vi "Magnetic Drift Correction (USE THIS ONE).vi"() -> ()   [LabVIEW 2025]
uses:
  <instrlib>/SMS LabVIEW Drivers/Source Code/Cryogenic Ltd SMSXXX.lvlib
  Downloads/Magnet Array.ctl
  <instrlib>/SMS LabVIEW Drivers/Source Code/Public/PSU Status.ctl
  Labview-File/QMH (STM Auto)/CTL's/Scan_Params (QMH).ctl
  Labview-File/Magnetic Drift Correction/XY_Coords(Final).ctl
panel:
  out "Current MID (T)":dbl
  out "Bias Iitial Y (m)":dbl
  out "Bias Initial X (m)":dbl
  in  "P-Mode Ramp Rate (A/s)":dbl=0.02
  out "Final coordinates (m)":cluster{"Xc":sgl, "Yc":sgl} {"Yc" format="%.4p"; "Xc" format="%.4p"}
  out "Initial coordinates (m)":cluster{"Xc":sgl, "Yc":sgl} {"Yc" format="%.4p"; "Xc" format="%.4p"}
  out "Translation (m)":T1
  out "Output (T)":dbl
  out "Initial MID (T)":dbl
  in  "Field Range":T2={"Sweep States"=enum."SET FIELD", "VISA Connection"="COM4", "Fields(T)"=[]}
  in  "Lead- Mode Ramp Rate (A/s)":dbl=0.02
  in  "Start":bool
  out "Errors":errorcluster[](array[cluster])
  in  "stop":bool
  out "Current Index":i32=1
  in  "Next Field":bool
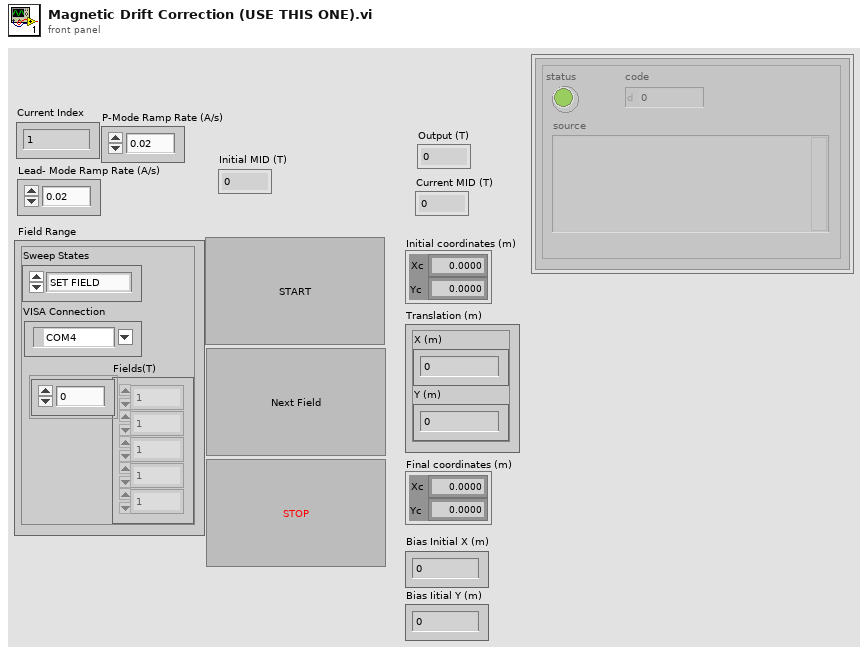
[diagram p1: front panel]
types:
  T1 = typedef "XY_Coords(Final).ctl" = cluster{"X (m)":dbl, "Y (m)":dbl}
  T2 = cluster{"Sweep States":enum16{"SET FIELD", "SWEEP IDLE", "NEXT FIELD", "SWEEP DONE"}, "VISA Connection":refnum<visa-resource-name>, "Fields(T)":dbl[]}
  T3 = enum16{"1. BIAS", "2. INIT_SCAN", "3. SCAN_IDLE", "4. INTER_SCAN", "5. NEW_COORDS_&_FRAME", "6. FINAL_SCAN", "7. POLL_BIAS", "8. Z-CONT.", "9. STOP"}
  T4 = enum16{"1. INIT MAG", "2. MAG ON", "3. MAG_STAB", "4. MAG IDLE", "5. PREP NEXT FIELD", "6. APPLY NEXT FIELD", "7. PREP OFF", "8. MAG OFF (Reset)"}
  T5 = typedef "Scan_Params (QMH).ctl" = cluster{"Setpoint (I)":dbl[], "Bias (V)":dbl[], "Number of scans":u8, "Port number (3364)":u32, "Avoid zero threshold (V)":dbl, "Current State":enum16{"1. BIAS", "2. INIT_SCAN", "3. SCAN_IDLE", "4. INTER_SCAN", "5. NEW_COORDS_&_FRAME", "6. FINAL_SCAN", "7. POLL BIAS", "8. Z-CONT", "9. STOP"}}
  T6 = typedef "Cryogenic Ltd SMSXXX.lvlib/PSU Status.ctl" = cluster{"Ramp Target":enum16{"ZERO", "MID", "MAX"}, "Pause":bool, "Switch Heater":bool, "Persistent Field":dbl, "Persistent Current":dbl, "Tesla":bool, "Output (T)":dbl, "Output (A)":dbl, "X Trip":enum16{"DISABLED", "ENABLED", "ACTIVE"}, "Ramp Rate (A/s)":dbl, "V Limit (V)":dbl, "Heater Voltage":dbl, "MAX Setpoint (A)":dbl, "MAX Setpoint (T)":dbl, "MID Setpoint (A)":dbl, "MID Setpoint (T)":dbl, "Lock":bool, "Field Constant":dbl, "Remote":bool, "Direction":enum16{"POSITIVE", "NEGATIVE", "OPEN", "UNIPOLAR"}, "Helium Level":u16, "Quench !":bool, "Voltage":dbl, "V Limit !":bool, "Ramping":bool, "At Target":bool, "Trip Field":dbl, "Trip Current":dbl, "Enum":enum16{"1. INIT MAG", "2. MAG ON ", "3. MAG_STAB", "4. MAG IDLE", "5. NEXT FIELD", "6. MAG OFF (Reset)"}}
  T7 = enum16{"SET FIELD", "SWEEP IDLE", "NEXT FIELD", "SWEEP DONE"}
  T8 = typedef "Magnet Array.ctl" = cluster{"Sweep States":enum16{"SET FIELD", "SWEEP IDLE", "NEXT FIELD", "SWEEP DONE"}, "VISA Connection":refnum<visa-resource-name>, "Fields(T)":dbl[]}
  T9 = typedef "Scan_Params (QMH).ctl" = cluster{"Setpoint (I)":dbl[], "Bias (V)":dbl[], "Number of scans":u8, "Port number (3364)":u32, "Avoid zero threshold (V)":dbl, "Current State":enum16{"1. BIAS", "2. INIT_SCAN", "3. SCAN_IDLE", "4. INTER_SCAN", "5. NEW_COORDS_&_FRAME", "6. FINAL_SCAN", "7. POLL_BIAS", "8. Z-CONT.", "9. STOP"}}
  T10 = enum16{"RAMP TO ZERO", "RAMP TO MID", "RAMP TO MAX"}
  T11 = typedef "PSU Status.ctl" = cluster{"Ramp Target":enum16{"ZERO", "MID", "MAX"}, "Pause":bool, "Switch Heater":bool, "Persistent Field":dbl, "Persistent Current":dbl, "Tesla":bool, "Output (T)":dbl, "Output (A)":dbl, "X Trip":enum16{"DISABLED", "ENABLED", "ACTIVE"}, "Ramp Rate (A/s)":dbl, "V Limit (V)":dbl, "Heater Voltage":dbl, "MAX Setpoint (A)":dbl, "MAX Setpoint (T)":dbl, "MID Setpoint (A)":dbl, "MID Setpoint (T)":dbl, "Lock":bool, "Field Constant":dbl, "Remote":bool, "Direction":enum16{"POSITIVE", "NEGATIVE", "OPEN", "UNIPOLAR"}, "Helium Level":u16, "Quench !":bool, "Voltage":dbl, "V Limit !":bool, "Ramping":bool, "At Target":bool, "Trip Field":dbl, "Trip Current":dbl, "Current State":enum16{"1. INIT MAG", "2. MAG ON", "3. MAG_STAB", "4. MAG IDLE", "5. PREP NEXT FIELD", "6. APPLY NEXT FIELD", "7. PREP OFF", "8. MAG OFF (Reset)"}, "MAG Reference":refnum<visa-resource-name>}
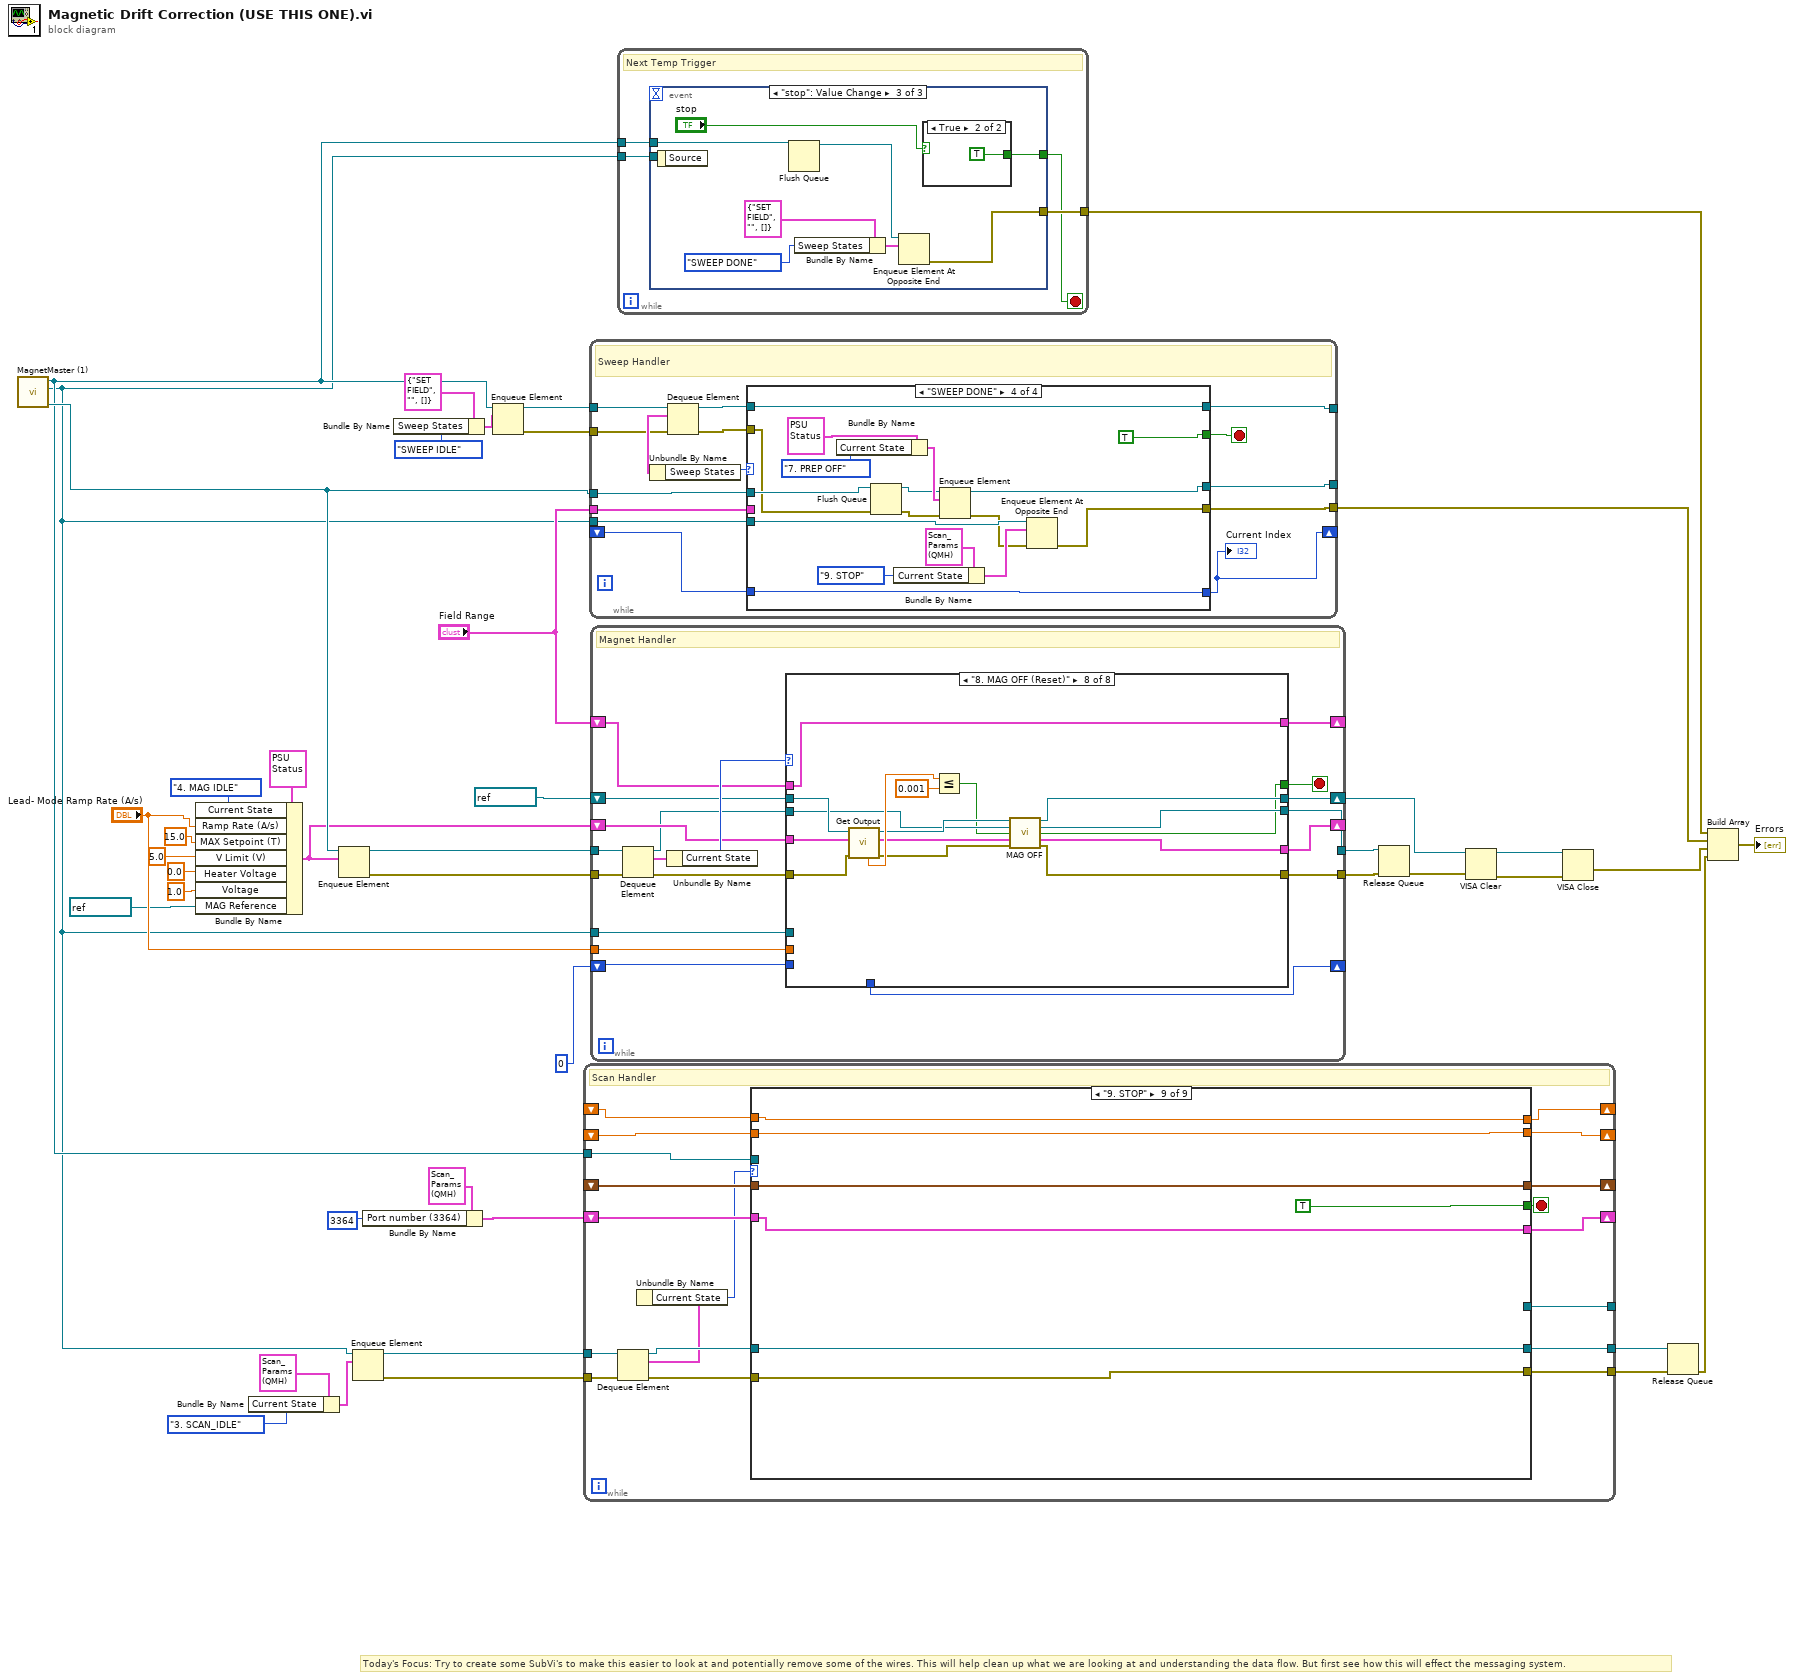
[diagram p0: block diagram]
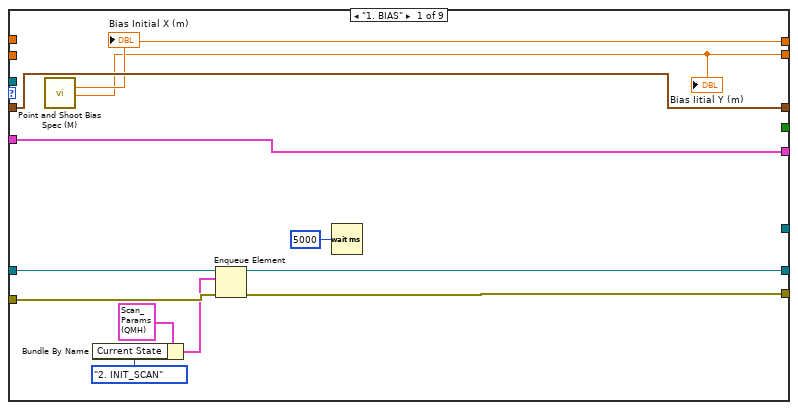
[diagram p2: hidden frame]
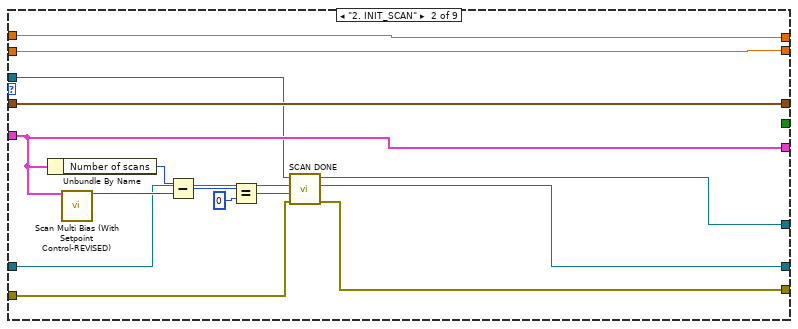
[diagram p3: hidden frame]
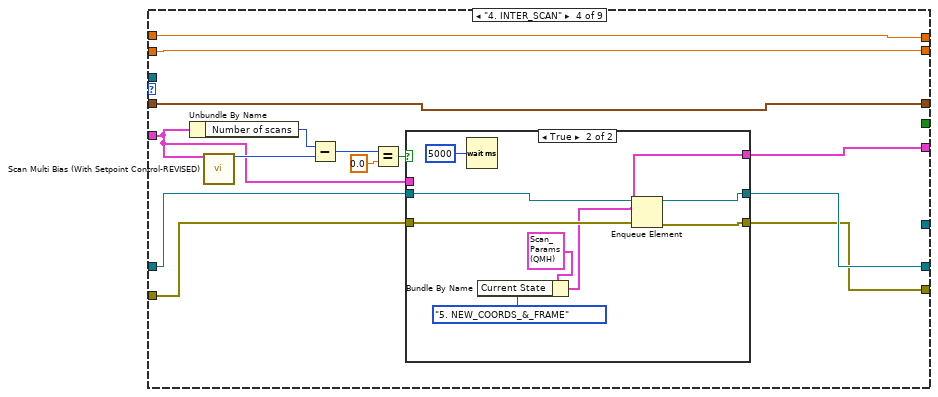
[diagram p5: hidden frame]
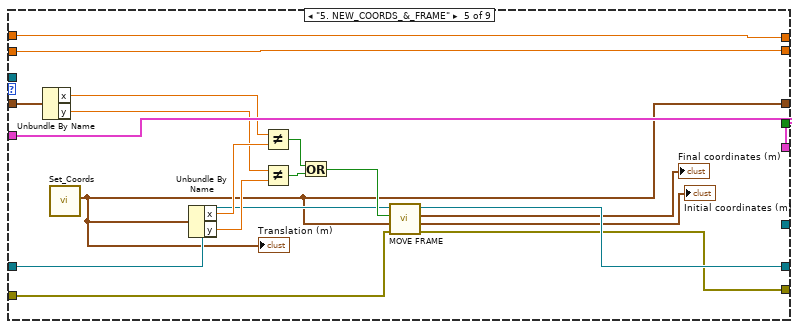
[diagram p7: hidden frame]
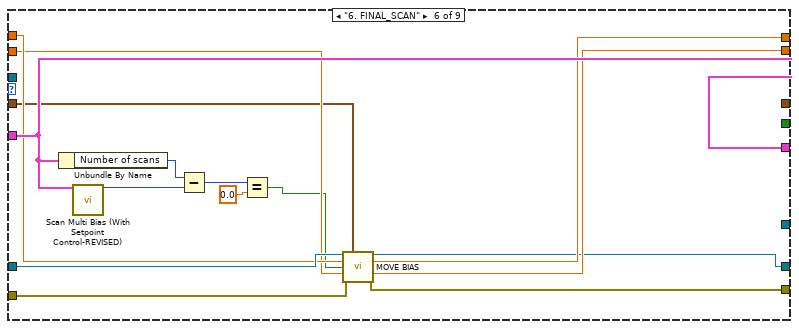
[diagram p8: hidden frame]
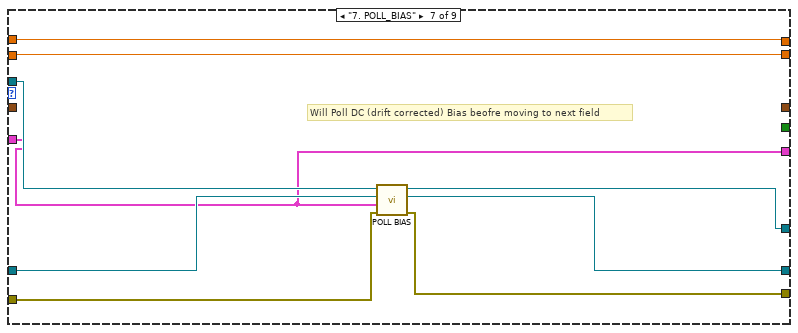
[diagram p9: hidden frame]
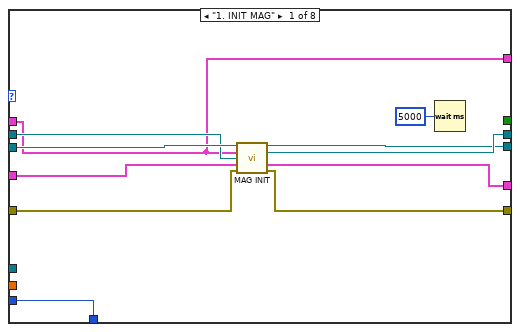
[diagram p11: hidden frame]
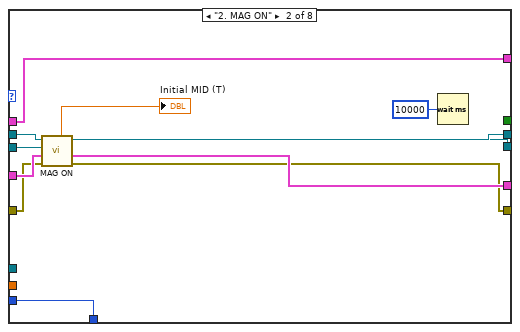
[diagram p12: hidden frame]
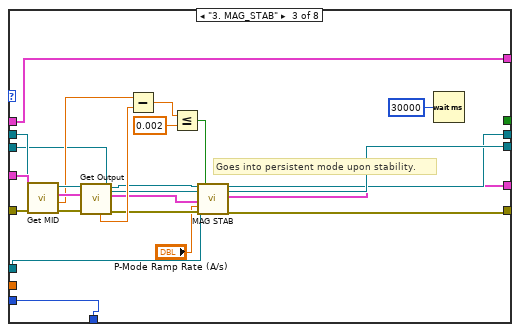
[diagram p13: hidden frame]
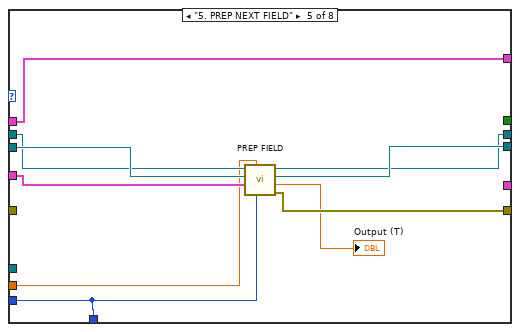
[diagram p15: hidden frame]
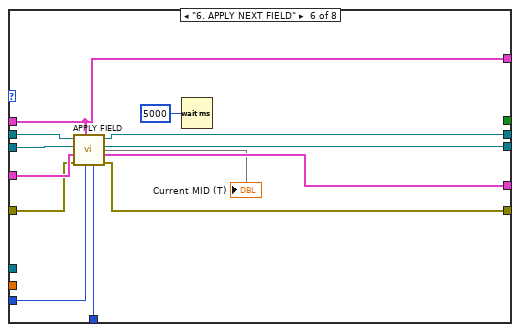
[diagram p16: hidden frame]
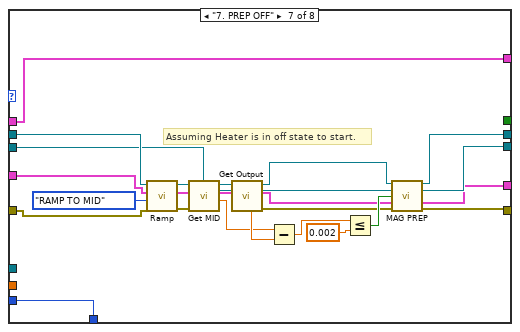
[diagram p17: hidden frame]
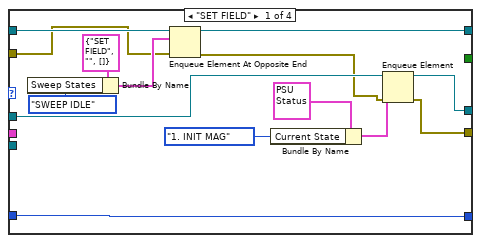
[diagram p18: hidden frame]
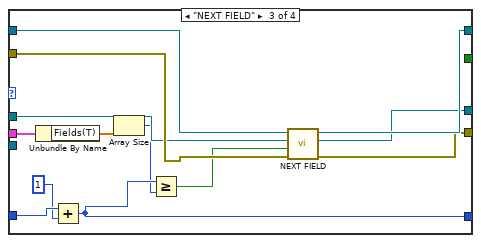
[diagram p20: hidden frame]
diagram:
  # "Today's Focus: Try to create some SubVi's to make this easier to look at and potentially remove some of the wires. This will help clean up what we are looking at and understanding the data flow. But first see how this will effect the messaging system."
  n1 = call "MagnetMaster (1).vi"() -> ("MaqQ"=w34:refnum<queue>, "ScanQ"=w3:refnum<queue>, "SweepQ"=w4:refnum<queue>)  [unwired: 9 in]
  n2 = Bundle By Name(cluster=T6 {"Ramp Target"=enum."ZERO", "Pause"=FALSE, "Switch Heater"=FALSE, "Persistent Field"=0.0, "Persistent Current"=0.0, "Tesla"=FALSE, "Output (T)"=0.0, "Output (A)"=0.0, "X Trip"=enum."DISABLED", "Ramp Rate (A/s)"=0.0, "V Limit (V)"=0.0, "Heater Voltage"=0.0, "MAX Setpoint (A)"=0.0, "MAX Setpoint (T)"=0.0, "MID Setpoint (A)"=0.0, "MID Setpoint (T)"=0.0, "Lock"=FALSE, "Field Constant"=0.0, "Remote"=FALSE, "Direction"=enum."POSITIVE", "Helium Level"=0, "Quench !"=FALSE, "Voltage"=0.0, "V Limit !"=FALSE, "Ramping"=FALSE, "At Target"=FALSE, "Trip Field"=0.0, "Trip Current"=0.0, "Enum"=enum."1. INIT MAG"} ("PSU Status In"), "Current State"=T4."4. MAG IDLE", "Ramp Rate (A/s)"="Lead- Mode Ramp Rate (A/s)", "MAX Setpoint (T)"=15.0, "V Limit (V)"=5.0, "Heater Voltage"=0.0, "Voltage"=1.0, "MAG Reference"=refnum<visa-resource-name> "COM4") -> (w30:T6)
  n3 = Bundle By Name(cluster=T5 {"Setpoint (I)"=[], "Bias (V)"=[], "Number of scans"=1, "Port number (3364)"=3364, "Avoid zero threshold (V)"=0.004999999888241291, "Current State"=enum."1. BIAS"} ("element"), "Current State"=T3."3. SCAN_IDLE") -> (w19:T5)
  n4 = Enqueue Element(queue=w34, element=w30) -> (queue out=w33:refnum<queue>, error out=w32:errorcluster)  [unwired: 2 in, 1 out]
  n5 = Enqueue Element(queue=w3, element=w19) -> (queue out=w21:refnum<queue>, error out=w20:errorcluster)  [unwired: 2 in, 1 out]
  n6 = Bundle By Name(cluster=T5 {"Setpoint (I)"=[], "Bias (V)"=[], "Number of scans"=1, "Port number (3364)"=3364, "Avoid zero threshold (V)"=0.004999999888241291, "Current State"=enum."1. BIAS"} ("element"), "Port number (3364)"=u32 3364) -> (w13:T5)
  n7 = Bundle By Name(cluster=T8 {"Sweep States"=enum."SET FIELD", "VISA Connection"="", "Fields(T)"=[]} ("element"), "Sweep States"=T7."SWEEP IDLE") -> (w37:T8)
  n8 = Enqueue Element(queue=w4, element=w37) -> (queue out=w39:refnum<queue>, error out=w35:errorcluster)  [unwired: 2 in, 1 out]
  n9 = while {
    tunnel: w20 -> [w54]
    shift-right: [w59] -> _
    shift-left: w13 -> [w62]
    tunnel: [w61] -> w17
    shift-right: [w58] -> _
    shift-left: _ -> [w57]
    tunnel: [w55] -> w16
    tunnel: w21 -> [w52]
    tunnel: w4 -> [w51]
    tunnel: [w50] -> _
    shift-right: [w44] -> _
    shift-left: _ -> [w46]
    shift-right: [w47] -> _
    shift-left: _ -> [w45]
    stop <- w56 stop-if-true
    # "Scan Handler"
    n10 = Dequeue Element(queue=w52, error in (no error)=w54) -> (queue out=w60:refnum<queue>, element=w48:T9, error out=w53:errorcluster)  [unwired: 1 in, 1 out]
    n11 = Unbundle By Name(w48) -> ("Current State"=w49:T3)
    n12 = case shown="\"9. STOP\"" w49 {
      tunnel: w62 -> [w72 w82 w93 w100 w137 w149 w153 w164 w170]
      tunnel: [w73 w83 w92 w102 w128 w138 w158 w163 w172] -> w61
      tunnel: w53 -> [w68 w85 _ w97 w125 w146 w159 w162 w171]
      tunnel: w60 -> [w74 w84 w92 w103 w129 w145 w160 w163 w172]
      tunnel: [w72 w82 w93 w101 w137 w149 w153 w164 w170] -> w59
      tunnel: [w71 w80 w94 w99 w122 _ _ _ w169] -> w58
      tunnel: w57 -> [w71 w80 w94 w99 w127 w139 _ _ w169]
      tunnel: [_ _ _ _ _ _ _ _ TRUE] -> w56
      tunnel: [w69 w79 _ w98 w126 w147 w157 w162 w171] -> w55
      tunnel: w51 -> [_ w78 _ _ _ _ w161 _ _]
      tunnel: [_ w77 _ _ _ _ w156 _ _] -> w50
      tunnel: [w65 w76 w91 w95 w120 w141 w155 w166 w168] -> w44
      tunnel: [w64 w75 w90 w96 w121 w140 w154 w165 w167] -> w47
      tunnel: w46 -> [_ w76 w91 w95 w120 w144 w155 w166 w168]
      tunnel: w45 -> [_ w75 w90 w96 w121 w143 w154 w165 w167]
      frame "1. BIAS" {
        n13 = call "Point and Shoot Bias Spec (M).vi"() -> ("Initial Y (m)"=w64:dbl, "Inital X (m)"=w65:dbl)  [unwired: 10 in]
        "Bias Initial X (m)" <- w65
        "Bias Iitial Y (m)" <- w64
        n14 = Bundle By Name(cluster=T5 {"Setpoint (I)"=[], "Bias (V)"=[], "Number of scans"=1, "Port number (3364)"=3364, "Avoid zero threshold (V)"=0.004999999888241291, "Current State"=enum."1. BIAS"} ("element"), "Current State"=T3."2. INIT_SCAN") -> (w66:T5)
        n15 = Enqueue Element(queue=w74, element=w66, error in (no error)=w68) -> (queue out=w73:refnum<queue>, error out=w69:errorcluster)  [unwired: 1 in, 1 out]
        n16 = Wait (ms)(milliseconds to wait=u32 5000) -> ()  [unwired: 1 out]
      }
      frame "2. INIT_SCAN" {
        n17 = Unbundle By Name(w82) -> ("Number of scans"=w81:u8)
        n18 = call "Scan Multi Bias (With Setpoint Control-REVISED).vi"("Scan Parameters"=w82) -> ("Scan"=w86:u8)  [unwired: 13 in, 1 out]
        n19 = Subtract(x=w81, y=w86) -> (x-y=w89:u8)
        n20 = Equal?(x=w89, y=u8 0) -> (x = y?=w87:bool)
        n21 = call "SCAN DONE.vi"("error in (no error)"=w85, "Boolean"=w87, "ScanQ in"=w84, "Queue in"=w78) -> ("error out"=w79:errorcluster, "ScanQ out"=w83:refnum<queue>, "Queue out"=w77:refnum<queue>)  [unwired: 5 in]
      }
      frame "3. SCAN_IDLE" {
      }
      frame "4. INTER_SCAN" {
        n22 = Unbundle By Name(w100) -> ("Number of scans"=w104:u8)
        n23 = call "Scan Multi Bias (With Setpoint Control-REVISED).vi"("Scan Parameters"=w100) -> ("Scan"=w105:u8)  [unwired: 13 in, 1 out]
        n24 = Subtract(x=w104, y=w105) -> (x-y=w107:u8)
        n25 = Equal?(x=w107, y=0.0) -> (x = y?=w106:bool)
        n26 = case shown="True" w106 {
          tunnel: w103 -> [w111 w118]
          tunnel: [w111 w117] -> w102
          tunnel: [w110 w113] -> w101
          tunnel: w100 -> [w110 _]
          tunnel: [w109 w116] -> w98
          tunnel: w97 -> [w109 w115]
          frame False {
          }
          frame True {
            n27 = Wait (ms)(milliseconds to wait=u32 5000) -> ()  [unwired: 1 out]
            n28 = Bundle By Name(cluster=T5 {"Setpoint (I)"=[], "Bias (V)"=[], "Number of scans"=1, "Port number (3364)"=3364, "Avoid zero threshold (V)"=0.004999999888241291, "Current State"=enum."2. INIT_SCAN"} ("element"), "Current State"=T3."5. NEW_COORDS_&_FRAME") -> (w113:T5)
            n29 = Enqueue Element(queue=w118, element=w113, error in (no error)=w115) -> (queue out=w117:refnum<queue>, error out=w116:errorcluster)  [unwired: 1 in, 1 out]
          }
        }
      }
      frame "5. NEW_COORDS_&_FRAME" {
        n30 = Unbundle By Name(w127) -> ("x"=w131:dbl, "y"=w130:dbl)
        n31 = call "Set_Coords.vi"() -> ("return value"=w122:cluster{"x":dbl, "y":dbl})  [unwired: 10 in, 1 out]
        "Translation (m)" <- w122
        n32 = Unbundle By Name(w122) -> ("x"=w134:dbl, "y"=w133:dbl)
        n33 = Not Equal?(x=w131, y=w134) -> (x != y?=w136:bool)
        n34 = Not Equal?(x=w130, y=w133) -> (x != y?=w135:bool)
        n35 = Or(x=w136, y=w135) -> (x .or. y?=w132:bool)
        n36 = call "MOVE FRAME.vi"("error in (no error)"=w125, "return value"=w122, "Boolean"=w132, "Queue in"=w129) -> ("error out"=w126:errorcluster, "Initial coordinates (m)"=→"Initial coordinates (m)":cluster{"Xc":sgl, "Yc":sgl}, "Final coordinates (m)"=→"Final coordinates (m)":cluster{"Xc":sgl, "Yc":sgl}, "Queue out"=w128:refnum<queue>)  [unwired: 4 in]
      }
      frame "6. FINAL_SCAN" {
        n37 = Unbundle By Name(w149) -> ("Number of scans"=w148:u8)
        n38 = call "Scan Multi Bias (With Setpoint Control-REVISED).vi"("Scan Parameters"=w149) -> ("Scan"=w150:u8)  [unwired: 13 in, 1 out]
        n39 = Subtract(x=w148, y=w150) -> (x-y=w151:u8)
        n40 = Equal?(x=w151, y=0.0) -> (x = y?=w142:bool)
        n41 = call "MOVE BIAS.vi"("ScanQ in"=w145, "return value"=w139, "Initial X"=w144, "Boolean"=w142, "Initial Y"=w143, "error in (no error)"=w146) -> ("ScanQ out"=w138:refnum<queue>, "FInal X (m)"=w141:sgl, "Final Y (m)"=w140:sgl, "error out"=w147:errorcluster)  [unwired: 6 in]
      }
      frame "7. POLL_BIAS" {
        # "Will Poll DC (drift corrected) Bias beofre moving to next field"
        n42 = call "POLL BIAS.vi"("error in (no error)"=w159, "element"=w153, "ScanQ in"=w160, "SweepQ in"=w161) -> ("error out"=w157:errorcluster, "ScanQ out"=w158:refnum<queue>, "SweepQ Out"=w156:refnum<queue>)  [unwired: 5 in]
      }
      frame "8. Z-CONT." {
      }
      frame "9. STOP" {
      }
    }
  }
  n43 = while {
    tunnel: w39 -> [w187]
    shift-right: [w174] -> _
    shift-left: _ -> [w185]
    tunnel: [w184] -> _
    tunnel: [w182] -> _
    tunnel: [w180] -> w28
    tunnel: w34 -> [w178]
    tunnel: w35 -> [w177]
    tunnel: "Field Range" -> [w176]
    tunnel: w3 -> [w175]
    stop <- w179 stop-if-true
    # "Sweep Handler"
    n44 = Dequeue Element(queue=w187, error in (no error)=w177) -> (queue out=w183:refnum<queue>, element=w186:T8, error out=w181:errorcluster)  [unwired: 1 in, 1 out]
    n45 = Unbundle By Name(w186) -> ("Sweep States"=w188:T7)
    n46 = case shown="\"SWEEP DONE\"" w188 {
      tunnel: w185 -> [w201 w203 w216 w232]
      tunnel: [w202 _ w209 w230] -> w184
      tunnel: w183 -> [w200 _ w214 w233]
      tunnel: [w201 w203 w206 w232] -> w174
      tunnel: [w199 _ w213 w233] -> w182
      tunnel: w181 -> [w194 _ w212 w219]
      tunnel: [w192 _ w211 w223] -> w180
      tunnel: [_ _ _ TRUE] -> w179
      tunnel: w178 -> [w198 _ w210 w221]
      tunnel: w176 -> [_ _ w208 _]
      tunnel: w175 -> [_ _ _ w226]
      frame "SET FIELD" {
        n47 = Bundle By Name(cluster=T8 {"Sweep States"=enum."SET FIELD", "VISA Connection"="", "Fields(T)"=[]} ("element"), "Sweep States"=T7."SWEEP IDLE") -> (w196:T8)
        n48 = Enqueue Element At Opposite End(queue=w200, element=w196, error in (no error)=w194) -> (queue out=w199:refnum<queue>, error out=w193:errorcluster)  [unwired: 1 in, 1 out]
        n49 = Bundle By Name(cluster=T6 {"Ramp Target"=enum."ZERO", "Pause"=FALSE, "Switch Heater"=FALSE, "Persistent Field"=0.0, "Persistent Current"=0.0, "Tesla"=FALSE, "Output (T)"=0.0, "Output (A)"=0.0, "X Trip"=enum."DISABLED", "Ramp Rate (A/s)"=0.0, "V Limit (V)"=0.0, "Heater Voltage"=0.0, "MAX Setpoint (A)"=0.0, "MAX Setpoint (T)"=0.0, "MID Setpoint (A)"=0.0, "MID Setpoint (T)"=0.0, "Lock"=FALSE, "Field Constant"=0.0, "Remote"=FALSE, "Direction"=enum."POSITIVE", "Helium Level"=0, "Quench !"=FALSE, "Voltage"=0.0, "V Limit !"=FALSE, "Ramping"=FALSE, "At Target"=FALSE, "Trip Field"=0.0, "Trip Current"=0.0, "Enum"=enum."1. INIT MAG"} ("PSU Status In"), "Current State"=T4."1. INIT MAG") -> (w190:T6)
        n50 = Enqueue Element(queue=w198, element=w190, error in (no error)=w193) -> (queue out=w202:refnum<queue>, error out=w192:errorcluster)  [unwired: 1 in, 1 out]
      }
      frame "SWEEP IDLE" {
      }
      frame "NEXT FIELD" {
        n51 = Unbundle By Name(w208) -> ("Fields(T)"=w207:dbl[])
        n52 = Add(x=w216, y=1) -> (x+y=w206:i32)
        n53 = Array Size(array=w207) -> (size(s)=w204:i32)
        n54 = Greater Or Equal?(x=w206, y=w204) -> (x >= y?=w205:bool)
        n55 = call "NEXT FIELD.vi"("error in (no error)"=w212, "Boolean"=w205, "MagQ in"=w210, "Queue in"=w214) -> ("error out"=w211:errorcluster, "MagQ out"=w209:refnum<queue>, "Queue out"=w213:refnum<queue>)  [unwired: 5 in]
      }
      frame "SWEEP DONE" {
        n56 = Bundle By Name(cluster=T6 {"Ramp Target"=enum."ZERO", "Pause"=FALSE, "Switch Heater"=FALSE, "Persistent Field"=0.0, "Persistent Current"=0.0, "Tesla"=FALSE, "Output (T)"=0.0, "Output (A)"=0.0, "X Trip"=enum."DISABLED", "Ramp Rate (A/s)"=0.0, "V Limit (V)"=0.0, "Heater Voltage"=0.0, "MAX Setpoint (A)"=0.0, "MAX Setpoint (T)"=0.0, "MID Setpoint (A)"=0.0, "MID Setpoint (T)"=0.0, "Lock"=FALSE, "Field Constant"=0.0, "Remote"=FALSE, "Direction"=enum."POSITIVE", "Helium Level"=0, "Quench !"=FALSE, "Voltage"=0.0, "V Limit !"=FALSE, "Ramping"=FALSE, "At Target"=FALSE, "Trip Field"=0.0, "Trip Current"=0.0, "Enum"=enum."1. INIT MAG"} ("PSU Status In"), "Current State"=T4."7. PREP OFF") -> (w228:T6)
        n57 = Flush Queue(queue=w221, error in (no error)=w219) -> (queue out=w220:refnum<queue>, error out=w218:errorcluster)  [unwired: 1 out]
        n58 = Bundle By Name(cluster=T5 {"Setpoint (I)"=[], "Bias (V)"=[], "Number of scans"=1, "Port number (3364)"=3364, "Avoid zero threshold (V)"=0.004999999888241291, "Current State"=enum."1. BIAS"} ("element"), "Current State"=T3."9. STOP") -> (w225:T5)
        n59 = Enqueue Element(queue=w220, element=w228, error in (no error)=w218) -> (queue out=w230:refnum<queue>, error out=w224:errorcluster)  [unwired: 1 in, 1 out]
        n60 = Enqueue Element At Opposite End(queue=w226, element=w225, error in (no error)=w224) -> (error out=w223:errorcluster)  [unwired: 1 in, 2 out]
      }
    }
    "Current Index" <- w174
  }
  n61 = while {
    tunnel: w33 -> [w251]
    tunnel: [w247] -> w42
    shift-right: [w246] -> _
    shift-left: w30 -> [w249]
    shift-right: [w245] -> w10
    shift-left: refnum<visa-resource-name> "COM4" ("MAG Reference") -> [w244]
    tunnel: [w243] -> w43
    tunnel: w32 -> [w242]
    shift-right: [w236] -> _
    shift-left: 0 -> [w240]
    tunnel: "Lead- Mode Ramp Rate (A/s)" -> [w238]
    tunnel: w3 -> [w237]
    shift-right: [w234] -> _
    shift-left: "Field Range" -> [w241]
    stop <- w235 stop-if-true
    # "Magnet Handler"
    n62 = Dequeue Element(queue=w251, error in (no error)=w242) -> (queue out=w239:refnum<queue>, element=w252:T11, error out=w248:errorcluster)  [unwired: 1 in, 1 out]
    n63 = Unbundle By Name(w252) -> ("Current State"=w250:T4)
    n64 = case "MAG STATE MACHINE" shown="\"8. MAG OFF (Reset)\"" w250 {
      tunnel: w249 -> [w259 w275 w298 w305 w313 w324 w350 w366]
      tunnel: w248 -> [w257 w273 w299 w304 _ w323 w349 w367]
      tunnel: [w262 w270 w279 w304 w310 w327 w332 w354] -> w247
      tunnel: [w260 w271 w280 w305 _ w320 w333 w357] -> w246
      tunnel: [w263 w272 w283 w303 w309 w321 w335 w358] -> w245
      tunnel: w244 -> [w255 w274 w297 w303 w312 w325 w351 w368]
      tunnel: [w261 w269 w284 w302 w315 w328 w334 w356] -> w243
      tunnel: w241 -> [w253 w264 w276 w300 w306 w317 w329 w353]
      tunnel: w240 -> [w254 w265 w277 w301 w307 w322 w330 _]
      tunnel: w239 -> [w258 w268 w288 w302 w314 w319 w331 w361]
      tunnel: w238 -> [_ _ _ _ w311 _ _ _]
      tunnel: w237 -> [_ _ w287 _ _ _ _ _]
      tunnel: [w254 w265 w277 w301 w307 w318 w330 _] -> w236
      tunnel: [_ _ _ _ _ _ _ w355] -> w235
      tunnel: [w253 w264 w276 w300 w306 w317 w329 w353] -> w234
      frame "1. INIT MAG" {
        n65 = call "MAG INIT.vi"("Queue in"=w258, "Field Range"=w253, "SMS VISA resource name IN"=w255, "PSU Status In"=w259, "error in (no error)"=w257) -> ("Queue out"=w261:refnum<queue>, "VISA Resource Name Out"=w263:refnum<visa-resource-name>, "PSU Status Out"=w260:T11, "error out"=w262:errorcluster)  [unwired: 7 in]
        n66 = Wait (ms)(milliseconds to wait=u32 5000) -> ()  [unwired: 1 out]
      }
      frame "2. MAG ON" {
        n67 = call "MAG ON.vi"("error in (no error)"=w273, "PSU Status In"=w275, "MagQ in"=w268, "VISA Refnum in"=w274) -> ("error out"=w270:errorcluster, "PSU Status Out"=w271:T6, "MagQ out"=w269:refnum<queue>, "VISA Refnum out"=w272:refnum<visa-resource-name>, "MID Setpoint (T)"=→"Initial MID (T)":dbl)  [unwired: 3 in]
        n68 = Wait (ms)(milliseconds to wait=u32 10000) -> ()  [unwired: 1 out]
      }
      frame "3. MAG_STAB" {
        # "Goes into persistent mode upon stability."
        n69 = call <instrlib>:"Get MID.vi"("Error in (no error)"=w299, "PSU Status In"=w298, "VISA Resource Name In"=w297) -> ("Error out"=w296:errorcluster, "MID Setpoint (T)"=w292:dbl, "PSU Status Out"=w295:T6, "VISA Resource Name Out"=w294:refnum<visa-resource-name>)  [unwired: 3 in, 2 out]
        n70 = call <instrlib>:"Get Output.vi"("Error in (no error)"=w296, "PSU Status In"=w295, "VISA Resource Name In"=w294) -> ("Error out"=w285:errorcluster, "PSU Status Out"=w286:T6, "VISA Resource Name Out"=w289:refnum<visa-resource-name>, "Output (T)"=w290:dbl)  [unwired: 3 in, 2 out]
        n71 = Subtract(x=w292, y=w290) -> (x-y=w291:dbl)
        n72 = Less Or Equal?(x=w291, y=0.002) -> (x <= y?=w282:bool)
        n73 = call "MAG STAB.vi"("VISA In"=w289, "MagQ"=w288, "ScanQ"=w287, "PSU Status In"=w286, "P-Mode Ramp Rate (A/s)"="P-Mode Ramp Rate (A/s)", "Error out"=w285, "Boolean"=w282) -> ("VISA Out"=w283:refnum<visa-resource-name>, "MagQ"=w284:refnum<queue>, "PSU Status Out"=w280:T6, "error out"=w279:errorcluster)  [unwired: 9 in]
        n74 = Wait (ms)(milliseconds to wait=u32 30000) -> ()  [unwired: 1 out]
      }
      frame "4. MAG IDLE" {
      }
      frame "5. PREP NEXT FIELD" {
        n75 = call "PREP FIELD.vi"("Numeric"=w307, "Lead- Mode Ramp Rate (A/s)"=w311, "PSU Status In"=w313, "MagQ in"=w314, "VISA Refnum in"=w312) -> ("error out"=w310:errorcluster, "Output (T)"=→"Output (T)":dbl, "MagQ out"=w315:refnum<queue>, "VISA Refnum out"=w309:refnum<visa-resource-name>)  [unwired: 3 in]
      }
      frame "6. APPLY NEXT FIELD" {
        n76 = call "APPLY FIELD.vi"("Numeric in"=w322, "Field and Tep  Range"=w317, "error in (no error)"=w323, "PSU Status In"=w324, "MagQ in"=w319, "VISA Refnum in"=w325) -> ("error out"=w327:errorcluster, "PSU Status Out"=w320:T6, "MagQ out"=w328:refnum<queue>, "VISA Refnum out"=w321:refnum<visa-resource-name>, 4:→"Current MID (T)", "Numeric out"=w318:i32)
        n77 = Wait (ms)(milliseconds to wait=u32 5000) -> ()  [unwired: 1 out]
      }
      frame "7. PREP OFF" {
        # "Assuming Heater is in off state to start."
        n78 = call <instrlib>:"Ramp.vi"("Error in (no error)"=w349, "Ramp Target"=T10."RAMP TO MID", "PSU Status In"=w350, "VISA Resource Name In"=w351) -> ("Error out"=w346:errorcluster, "PSU Status Out"=w347:T6, "VISA Resource Name Out"=w348:refnum<visa-resource-name>)  [unwired: 4 in, 1 out]
        n79 = call <instrlib>:"Get MID.vi"("Error in (no error)"=w346, "PSU Status In"=w347, "VISA Resource Name In"=w348) -> ("MID Setpoint (T)"=w340:dbl, "PSU Status Out"=w344:T6, "VISA Resource Name Out"=w345:refnum<visa-resource-name>)  [unwired: 3 in, 3 out]
        n80 = call <instrlib>:"Get Output.vi"("PSU Status In"=w344, "VISA Resource Name In"=w345) -> ("Error out"=w336:errorcluster, "PSU Status Out"=w337:T6, "VISA Resource Name Out"=w339:refnum<visa-resource-name>, "Output (T)"=w341:dbl)  [unwired: 4 in, 2 out]
        n81 = Subtract(x=w340, y=w341) -> (x-y=w343:dbl)
        n82 = Less Or Equal?(x=w343, y=0.002) -> (x <= y?=w338:bool)
        n83 = call "MAG PREP.vi"("VISA In"=w339, "MagQ"=w331, "Boolean"=w338, "PSU Status In"=w337, "Error In"=w336) -> ("VISA Out"=w335:refnum<visa-resource-name>, "MagQ"=w334:refnum<queue>, "PSU Status Out"=w333:T6, "error out"=w332:errorcluster)  [unwired: 7 in]
      }
      frame "8. MAG OFF (Reset)" {
        n84 = call <instrlib>:"Get Output.vi"("Error in (no error)"=w367, "PSU Status In"=w366, "VISA Resource Name In"=w368) -> ("Error out"=w360:errorcluster, "PSU Status Out"=w362:T6, "VISA Resource Name Out"=w363:refnum<visa-resource-name>, "Output (T)"=w365:dbl)  [unwired: 3 in, 2 out]
        n85 = Less Or Equal?(x=w365, y=0.001) -> (x <= y?=w359:bool)
        n86 = call "MAG OFF.vi"("VISA Resource Name Out"=w363, "MagQ"=w361, "Boolean"=w359, "PSU Status Out"=w362, "Error out"=w360) -> ("VISA Resource Name Out 2"=w358:refnum<visa-resource-name>, "MagQ 2"=w356:refnum<queue>, "Boolean 2"=w355:bool, "PSU Status Out 2"=w357:T6, "error out"=w354:errorcluster)  [unwired: 6 in]
      }
    }
  }
  n87 = while {
    tunnel: w4 -> [w372]
    tunnel: [w371] -> w29
    tunnel: w3 -> [w369]
    stop <- w370 stop-if-true
    # "Next Temp Trigger"
    n88 = event shown="[2] \"stop\": Value Change" {
      selector: _ -> [_ _ _]
      dyn-events: _ -> [_ _ _]
      timeout: _ -> [_ _ _]
      tunnel: w372 -> [w377 _ w384]
      tunnel: [w376 w382 w387] -> w371
      tunnel: [_ _ w385] -> w370
      tunnel: w369 -> [_ w380 _]
      event "Next Field": Value Change {
        n89 = event-data() -> ()  [unwired: 1 in, 1 out]
        n90 = Bundle By Name(cluster=T8 {"Sweep States"=enum."SET FIELD", "VISA Connection"="", "Fields(T)"=[]} ("element"), "Sweep States"=T7."NEXT FIELD") -> (w374:T8)
        n91 = Enqueue Element(queue=w377, element=w374) -> (error out=w376:errorcluster)  [unwired: 2 in, 2 out]
      }
      event "Start": Value Change {
        n92 = event-data() -> ()  [unwired: 1 in, 6 out]
        n93 = Bundle By Name(cluster=T5 {"Setpoint (I)"=[], "Bias (V)"=[], "Number of scans"=1, "Port number (3364)"=3364, "Avoid zero threshold (V)"=0.004999999888241291, "Current State"=enum."1. BIAS"} ("element"), "Current State"=T3."1. BIAS") -> (w379:T5)
        n94 = Enqueue Element(queue=w380, element=w379) -> (error out=w382:errorcluster)  [unwired: 2 in, 2 out]
      }
      event "stop": Value Change {
        n95 = event-data() -> ()  [unwired: 1 in, 1 out]
        n96 = Flush Queue(queue=w384) -> (queue out=w383:refnum<queue>)  [unwired: 1 in, 2 out]
        n97 = Bundle By Name(cluster=T8 {"Sweep States"=enum."SET FIELD", "VISA Connection"="", "Fields(T)"=[]} ("element"), "Sweep States"=T7."SWEEP DONE") -> (w389:T8)
        n98 = Enqueue Element At Opposite End(queue=w383, element=w389) -> (error out=w387:errorcluster)  [unwired: 2 in, 2 out]
        n99 = case shown="True" "stop" {
          tunnel: [FALSE ("stop 2") TRUE ("stop 2")] -> w385
          frame False {
          }
          frame True {
          }
        }
      }
    }
  }
  n100 = Release Queue(queue=w43, error in (no error)=w42) -> (error out=w9:errorcluster)  [unwired: 1 in, 2 out]
  n101 = VISA Clear(VISA resource name=w10, error in (no error)=w9) -> (VISA resource name out=w8:refnum<visa-resource-name>, error out=w7:errorcluster)
  n102 = VISA Close(VISA resource name=w8, error in (no error)=w7) -> (error out=w41:errorcluster)
  n103 = Release Queue(queue=w17, error in (no error)=w16) -> (error out=w15:errorcluster)  [unwired: 1 in, 2 out]
  n104 = Build Array(w29, w28, w41, w15) -> (→"Errors":errorcluster[])
